vi "Web Redirect Parameter Parser.vi"(0 "redirect URL":string="Return_Success.httml", 1 "Device":T1, 3 "error in (no error)":errorcluster) -> (7 "Output String":string, 10 "error out":errorcluster)   [LabVIEW 2016]
uses:
  Device Info.ctl
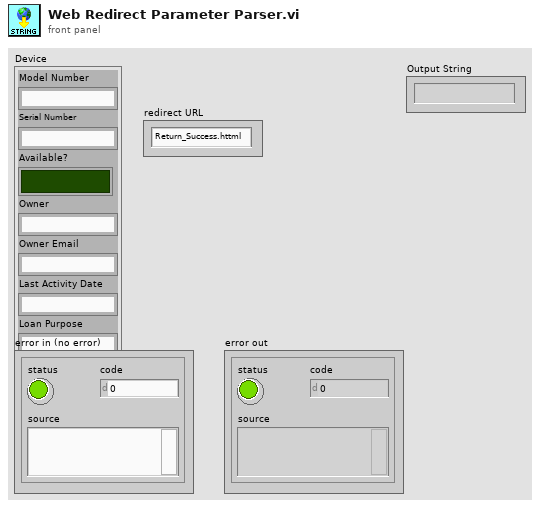
[diagram p1: front panel]
types:
  T1 = typedef "Device Info.ctl" = cluster{"Model Number":string, "Serial Number":string, "Available?":bool, "Owner":string, "Owner Email":string, "Last Activity Date":string, "Loan Purpose":string}
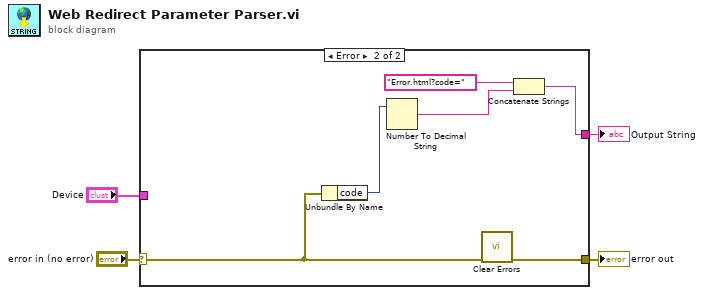
[diagram p0: block diagram]
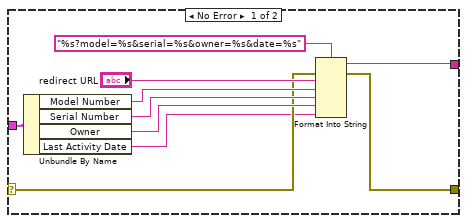
[diagram p2: hidden frame]
diagram:
  n1 = case shown="Error" "error in (no error)" {
    selector: "error in (no error)" -> [w7 w19]
    tunnel: [w6 w20] -> w3
    tunnel: "Device" -> [w14 _]
    tunnel: [w8 w15] -> w1
    frame No Error {
      n2 = Unbundle By Name(w14) -> ("Model Number"=w11:string, "Serial Number"=w10:string, "Owner"=w9:string, "Last Activity Date"=w5:string)
      n3 = Format Into String(format string="%s?model=%s&serial=%s&owner=%s&date=%s" ("initial string"), error in=w7, "redirect URL", w11, w10, w9, w5) -> (resulting string=w8:string, error out=w6:errorcluster)  [unwired: 1 in]
    }
    frame Error {
      n4 = Unbundle By Name(w19) -> ("code"=w18:i32)
      n5 = Number To Decimal String(number=w18) -> (decimal integer string=w16:string)  [unwired: 1 in]
      n6 = call <vilib>:"Clear Errors.vi"("error in (no error)"=w19) -> ("error out"=w20:errorcluster)  [unwired: 5 in, 1 out]
      n7 = Concatenate Strings("Error.html?code=", w16) -> (w15:string)
    }
  }
  "error out" <- w3
  "Output String" <- w1
